vi "Error Event.vi"(8 "error in (no error)":errorcluster, 11 "Command Handler in":refnum<class "Command Handler.lvclass">) -> (0 "error out":errorcluster)   [LabVIEW 2017, in "Command Handler.lvlib" / "Command Handler.lvclass"]
uses:
  Command Handler.lvclass
  Command Handler.lvclass/Command Handler.ctl
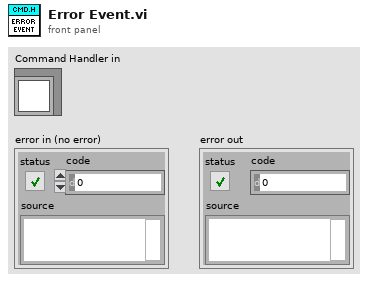
[diagram p1: front panel]
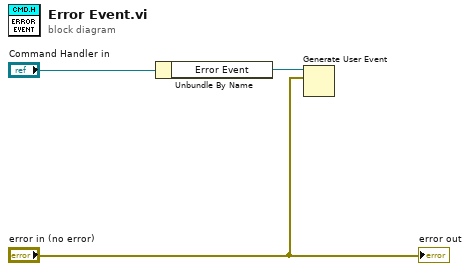
[diagram p0: block diagram]
diagram:
  n1 = Unbundle By Name("Command Handler in") -> ("Error Event"=w3:refnum<user-event>)
  n2 = Generate User Event(user event=w3, event data cluster="error in (no error)") -> ()  [unwired: 2 in, 2 out]
  "error out" <- "error in (no error)"
